vi "Read Analogue.vi"(8 "error in (no error)":errorcluster, 11 "Voltage Input in":refnum<class "Sim ACIR.lvclass">) -> (0 "error out":errorcluster, 2 "Measurement":dbl format="%.5f", 3 "Voltage Input out":refnum<class "Sim ACIR.lvclass">)   [LabVIEW 2021, in "Concrete.lvlib" / "Sim ACIR.lvclass"]
uses:
  Sim ACIR.lvclass
  <vilib>/numeric/Random Number (Range) DBL.vi
  Harware Abstraction/ACIR/ACIR.lvclass
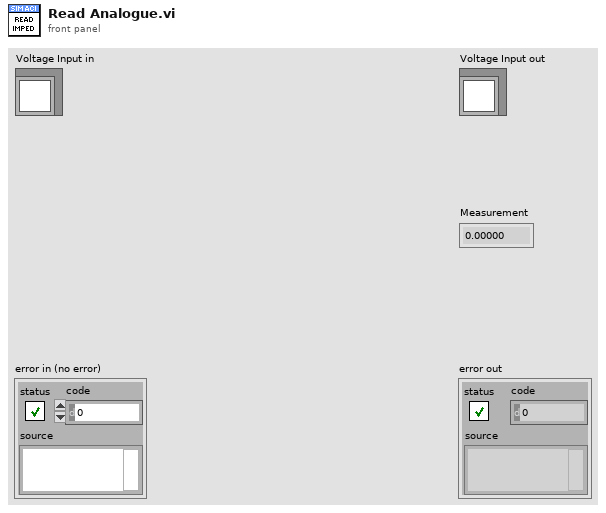
[diagram p1: front panel]
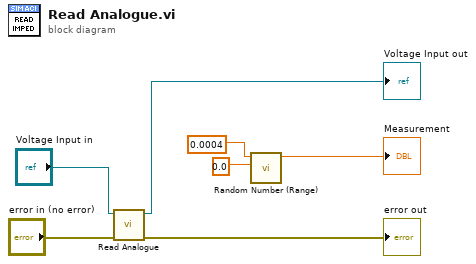
[diagram p0: block diagram]
diagram:
  n1 = call-parent "Read Analogue.vi"("error in (no error)"="error in (no error)", "PS in"="Voltage Input in") -> ("error out"=→"error out":errorcluster, "PS out"=→"Voltage Input out":refnum<class "Sim ACIR.lvclass">)  [unwired: 7 in, 1 out]
  n2 = call-poly <vilib>:"Random Number (Range).vi"("lower bound (0)"=0.0, "upper bound (100)"=0.0004) -> ("number"=→"Measurement":dbl)  [unwired: 9 in]
